vi "P-541 Test Panel.vi"() -> ()   [LabVIEW 2020]
panel:
  out "Diff":dbl
  in  "Position":dbl
  in  "Axis Name":string
  in  "Chassis Name":string
  in  "Wait for Reply":bool=TRUE
  out "Bool":bool
  out "Value":dbl
  out "Cmd Success":bool
  out "Connected":bool
  out "Waiting for Reply":bool
  out "Last Error":errorcluster
  out "Command History":string
  out "Reply":string
  in  "Command":string
  in  "Quit":bool
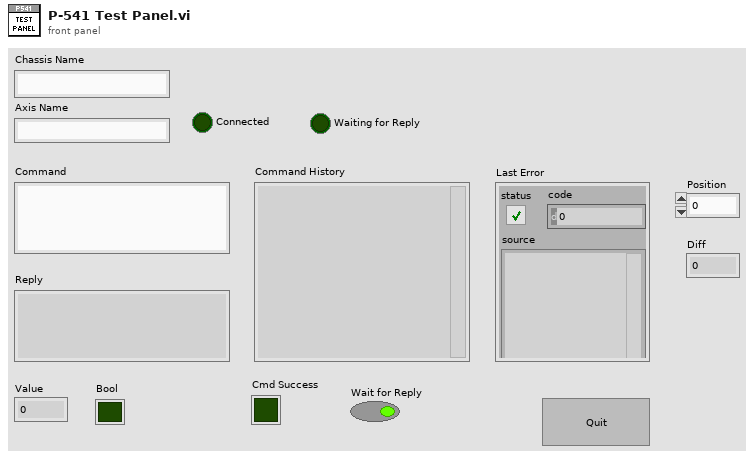
[diagram p1: front panel]
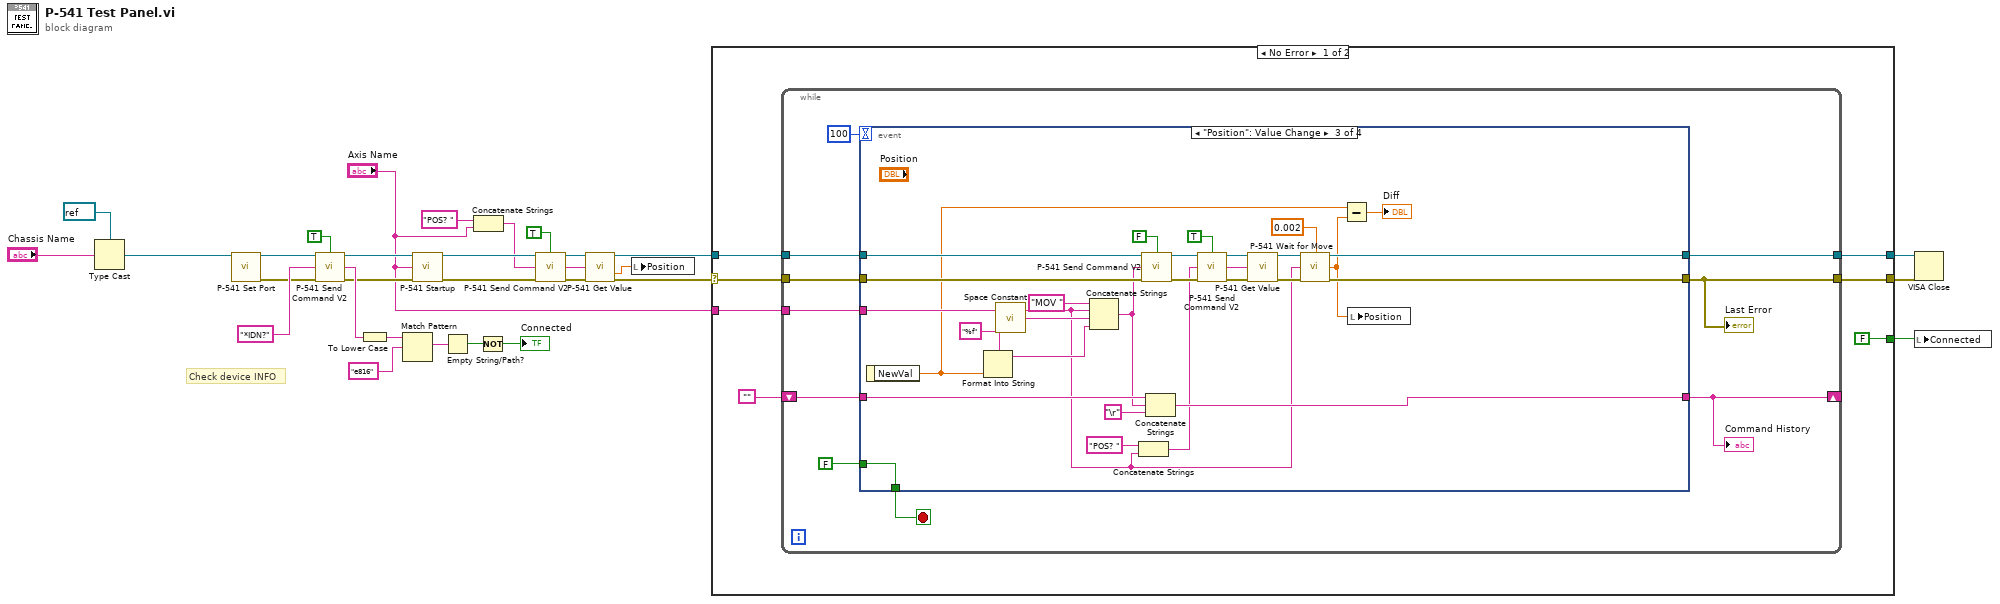
[diagram p0: block diagram]
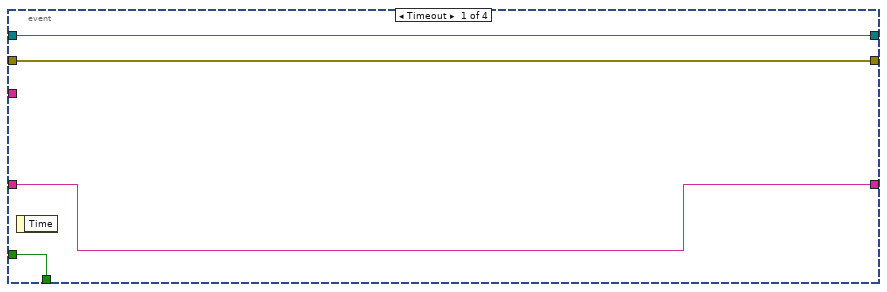
[diagram p2: hidden frame]
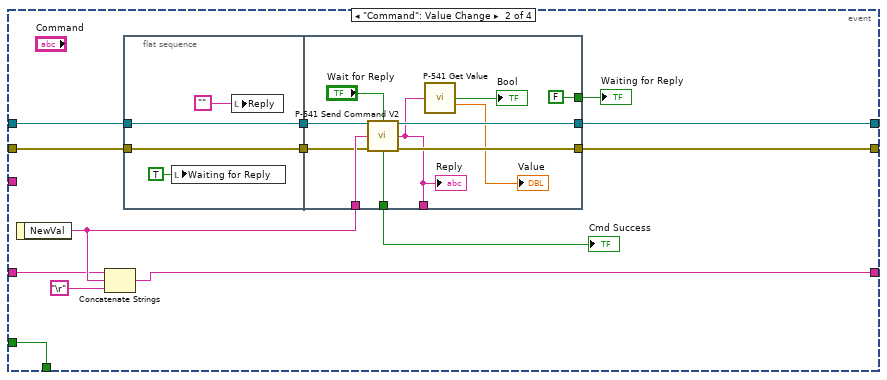
[diagram p3: hidden frame]
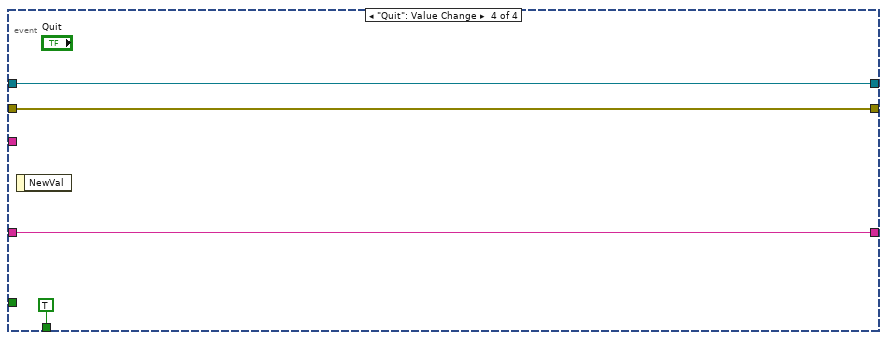
[diagram p4: hidden frame]
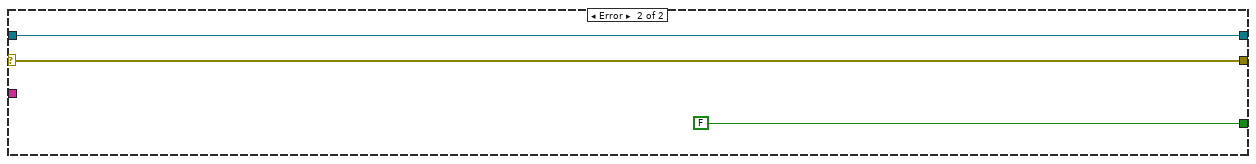
[diagram p5: hidden frame]
diagram:
  # "Check device INFO"
  n1 = Type Cast(type=refnum<visa-resource-name> refnum ("reference out"), x="Chassis Name") -> (*(type *) &x=w17:refnum<visa-resource-name>)
  n2 = call "P-541 Set Port.vi"("VISA Ref In"=w17) -> ("VISA Ref Out"=w16:refnum<visa-resource-name>, "Error Out"=w15:errorcluster)  [unwired: 13 in]
  n3 = call "P-541 Send Command V2.vi"("VISA Ref"=w16, "Wait for Reply (T)"=TRUE ("Wait for Reply?"), "Command"="*IDN?" ("string"), "Error In"=w15) -> ("VISA Ref Dup"=w14:refnum<visa-resource-name>, "Reply"=w25:string, "Error Out"=w13:errorcluster)  [unwired: 8 in, 1 out]
  n4 = To Lower Case(string=w25) -> (all lower case string=w27:string)
  n5 = Match Pattern(string=w27, regular expression="e816" ("string")) -> (match substring=w22:string)  [unwired: 1 in, 3 out]
  n6 = call "P-541 Startup.vi"("VISA Ref"=w14, "Axis Name"="Axis Name", "Error In"=w13) -> ("VISA Ref Out"=w12:refnum<visa-resource-name>, "Error Out"=w11:errorcluster)  [unwired: 11 in]
  n7 = Empty String/Path?(string/path=w22) -> (empty?=w24:bool)
  n8 = Concatenate Strings("POS? ", "Axis Name") -> (w9:string)
  n9 = Not(x=w24) -> (.not. x?=→"Connected":bool)
  n10 = call "P-541 Send Command V2.vi"("VISA Ref"=w12, "Wait for Reply (T)"=TRUE, "Command"=w9, "Error In"=w11) -> ("VISA Ref Dup"=w6:refnum<visa-resource-name>, "Reply"=w5:string, "Error Out"=w7:errorcluster)  [unwired: 8 in, 1 out]
  n11 = call "P-541 Get Value.vi"("VISA Pass Thru"=w6, "Cmd Reply"=w5, "Error In"=w7) -> ("VISA Ref Dup"=w4:refnum<visa-resource-name>, "Value"=w2:dbl, "Error Out"=w3:errorcluster)  [unwired: 9 in, 1 out]
  n12 = local write "Position"(w2) -> ()
  n13 = case shown="No Error" w3 {
    selector: w3 -> [w36 w114]
    tunnel: w4 -> [w37 w115]
    tunnel: [w35 w115] -> w30
    tunnel: [w34 w114] -> w29
    tunnel: [FALSE FALSE] -> w28
    tunnel: "Axis Name" -> [w31 _]
    frame No Error {
      n14 = while {
        tunnel: w37 -> [w45]
        tunnel: w36 -> [w44]
        tunnel: [w43] -> w35
        tunnel: [w41] -> w34
        shift-right: [w39] -> _
        shift-left: "" -> [w42]
        tunnel: w31 -> [w38]
        stop <- w46 stop-if-true
        n15 = event shown="[2] \"Position\": Value Change" {
          selector: _ -> [_ _ _ _]
          dyn-events: _ -> [_ _ _ _]
          timeout: 100 -> [_ _ _ _]
          tunnel: FALSE -> [w51 w64 w108 _]
          tunnel: [w51 w64 w108 TRUE] -> w46
          tunnel: w45 -> [w49 w63 w107 w112]
          tunnel: w44 -> [w48 w62 w106 w111]
          tunnel: [w49 w58 w84 w112] -> w43
          tunnel: [w48 w59 w83 w111] -> w41
          tunnel: w42 -> [w50 w55 w104 w109]
          tunnel: [w50 w54 w97 w109] -> w39
          tunnel: w38 -> [_ _ w85 _]
          event Timeout {
            n16 = event-data() -> ()  [unwired: 1 in, 1 out]
          }
          event "Command": Value Change {
            n17 = event-data() -> ("NewVal"=w57:string)  [unwired: 1 in]
            n18 = Concatenate Strings(w55, w57, "\r") -> (w54:string)
            n19 = flat-sequence {
              tunnel: w62 -> [w67]
              tunnel: w63 -> [w68]
              tunnel: [w68] -> w61
              tunnel: [w67] -> w60
              tunnel: w57 -> [w78]
              tunnel: w61 -> [w79]
              tunnel: w60 -> [w77]
              tunnel: [w76] -> w59
              tunnel: [w75] -> w58
              tunnel: [FALSE] -> w53
              tunnel: [w72] -> w52
              tunnel: [w69] -> _
              frame #0 {
                n20 = local write "Waiting for Reply"(TRUE ("Waiting for Cmd")) -> ()
                n21 = local write "Reply"("") -> ()
              }
              frame #1 {
                n22 = call "P-541 Send Command V2.vi"("VISA Ref"=w79, "Wait for Reply (T)"="Wait for Reply", "Command"=w78, "Error In"=w77) -> ("VISA Ref Dup"=w75:refnum<visa-resource-name>, "Reply"=w69:string, "Cmd Success"=w72:bool, "Error Out"=w76:errorcluster)  [unwired: 8 in]
                "Reply" <- w69
                n23 = call "P-541 Get Value.vi"("Cmd Reply"=w69) -> ("Bool"=→"Bool":bool, "Value"=→"Value":dbl)  [unwired: 11 in, 2 out]
              }
            }
            "Waiting for Reply" <- w53
            "Cmd Success" <- w52
          }
          event "Position": Value Change {
            n24 = event-data() -> ("NewVal"=w82:dbl)  [unwired: 1 in]
            n25 = Format Into String(format string="%f", w82) -> (resulting string=w100:string)  [unwired: 2 in, 1 out]
            n26 = call <vilib>:"Space Constant.vi"() -> ("String"=w102:string)
            n27 = Concatenate Strings("MOV ", w85, w102, w100) -> (w98:string)
            n28 = Concatenate Strings("POS? ", w85) -> (w89:string)
            n29 = call "P-541 Send Command V2.vi"("VISA Ref"=w107, "Wait for Reply (T)"=FALSE, "Command"=w98, "Error In"=w106) -> ("VISA Ref Dup"=w91:refnum<visa-resource-name>, "Error Out"=w90:errorcluster)  [unwired: 8 in, 2 out]
            n30 = Concatenate Strings(w104, w98, "\r") -> (w97:string)
            n31 = call "P-541 Send Command V2.vi"("VISA Ref"=w91, "Wait for Reply (T)"=TRUE, "Command"=w89, "Error In"=w90) -> ("VISA Ref Dup"=w93:refnum<visa-resource-name>, "Reply"=w94:string, "Error Out"=w95:errorcluster)  [unwired: 8 in, 1 out]
            n32 = call "P-541 Get Value.vi"("VISA Pass Thru"=w93, "Cmd Reply"=w94, "Error In"=w95) -> ("VISA Ref Dup"=w87:refnum<visa-resource-name>, "Error Out"=w86:errorcluster)  [unwired: 9 in, 2 out]
            n33 = call "P-541 Wait for Move.vi"("VISA Ref"=w87, "Threshold"=0.002, "Axis Name"=w85, "Error In"=w86) -> ("VISA Ref Dup"=w84:refnum<visa-resource-name>, "Position"=w81:dbl, "Error Out"=w83:errorcluster)  [unwired: 9 in]
            n34 = Subtract(x=w82, y=w81) -> (x-y=→"Diff":dbl)
            n35 = local write "Position"(w81) -> ()
          }
          event "Quit": Value Change {
            n36 = event-data() -> ()  [unwired: 1 in, 1 out]
          }
        }
        "Last Error" <- w41
        "Command History" <- w39
      }
    }
    frame Error {
    }
  }
  n37 = VISA Close(VISA resource name=w30, error in (no error)=w29) -> ()  [unwired: 1 out]
  n38 = local write "Connected"(w28) -> ()
